vi "Stop Core.vi"(10 "final error code":i32, 11 "ArduinoTranslationStage in":refnum<class "ArduinoTranslationStage.lvclass">) -> (3 "ArduinoTranslationStage out":refnum<class "ArduinoTranslationStage.lvclass">)   [LabVIEW 2023, in "ArduinoTranslationStage.lvlib" / "ArduinoTranslationStage.lvclass"]
doc: "<p>(<strong>Filename</strong>: <span class=\"dnl\">Actor Framework.lvlib:Actor.lvclass:Stop Core.vi</span>)</p>\n<p>Defines what the actor does before it stops. Use the <strong>final error code</strong> input to determine whether the actor shut down in response to an error.</p>\n<p>By default, this method passes the Stop message along to all <a href=\"nihelplauncher://docs/csh?context=lvcore_lvcomm_af_launch_nested_actor\">auto-stop nested actors</a>. A descendant class may override this method to define additional behavior, such as shutting down any processes the actor initiated in its override of the <a href=\"nihelplauncher://docs/csh?context=lvcore_lvcomm_af_actor_core\">Actor Core</a> method.</p>"
uses:
  ArduinoTranslationStage.lvclass
  <vilib>/ActorFramework/Actor/Actor.lvclass
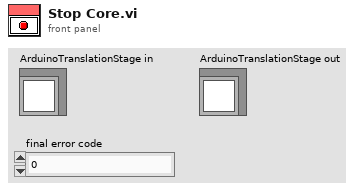
[diagram p1: front panel]
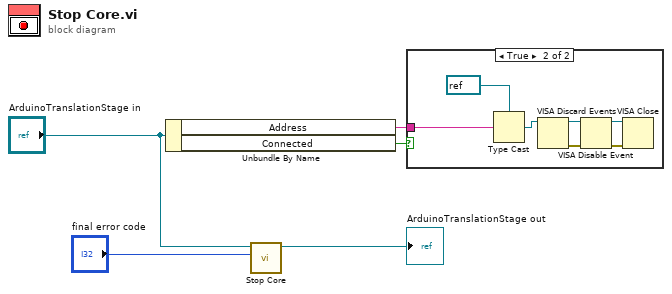
[diagram p0: block diagram]
diagram:
  n1 = Unbundle By Name("ArduinoTranslationStage in") -> ("Address"=w2:string, "Connected"=w1:bool)
  n2 = call-parent "Stop Core.vi"("final error code"="final error code", "Actor in"="ArduinoTranslationStage in") -> ("Actor out"=→"ArduinoTranslationStage out":refnum<class "ArduinoTranslationStage.lvclass">)  [unwired: 9 in]
  n3 = case shown="True" w1 {
    tunnel: w2 -> [_ w12]
    frame False {
    }
    frame True {
      n4 = Type Cast(type=refnum<visa-resource-name> refnum ("VISA resource name"), x=w12) -> (*(type *) &x=w10:refnum<visa-resource-name>)
      n5 = VISA Discard Events(11:w10) -> (0:w6:errorcluster, 3:w9:refnum<visa-resource-name>)  [unwired: 3 in]
      n6 = VISA Disable Event(8:w6, 11:w9) -> (0:w7:errorcluster, 3:w8:refnum<visa-resource-name>)  [unwired: 2 in]
      n7 = VISA Close(VISA resource name=w8, error in (no error)=w7) -> ()  [unwired: 1 out]
    }
  }
